vi "_Core(client).vi"(0 "XML config File Path":path=path "D:/work/Project support in lanzhou/OPCUA XML/xml/server config.xml", 1 "Server IP":string, 2 "client cert path(empty path)":path, 3 "timeout (5000 ms)":u32=5000, 4 "username/password":cluster{"username":string, "password":string}, 7 "error in (no error)":errorcluster, 9 "Op":T1) -> (8 "OPC UA data change event":refnum<user-event>, 10 "trusted Server certfications":path[](array[path]), 12 "server endpoint URL":string, 20 "OPC UA client refnum out":refnum<k21>, 27 "error out":errorcluster)   [LabVIEW 2014, in "OCPUA Client(UtilityMode).lvlib"]
uses:
  OCPUA Client(UtilityMode).lvlib
  _op(client).ctl
  <vilib>/OPCUA/NI OPC UA Client.lvlib
  OPCUA XML/OPCUA XML.lvlib
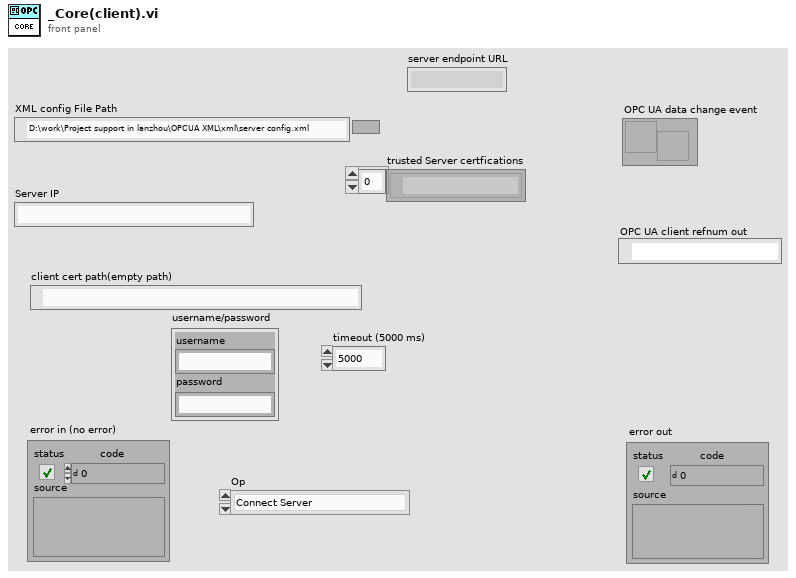
[diagram p1: front panel]
types:
  T1 = typedef "OCPUA Client(UtilityMode).lvlib/_op(client).ctl" = enum16{"Connect Server", "Get Client Refnum", "Disconnect Server"}
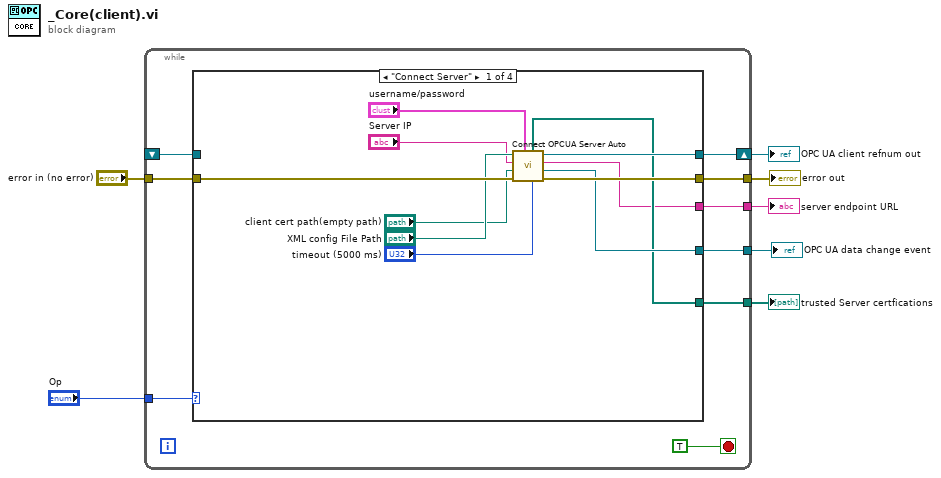
[diagram p0: block diagram]
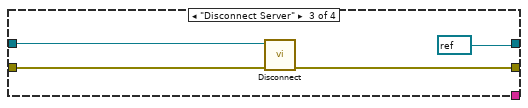
[diagram p3: hidden frame]
diagram:
  n1 = while {
    tunnel: "Op" -> [w15]
    shift-right: [w13] -> w4
    shift-left: _ -> [w14]
    tunnel: [w12] -> w5
    tunnel: "error in (no error)" -> [w11]
    tunnel: [w10] -> w3
    tunnel: [w9] -> w2
    tunnel: [w8] -> w1
    stop <- TRUE stop-if-true
    n2 = case shown="\"Connect Server\"" w15 {
      tunnel: w14 -> [_ w29 w31 w35]
      tunnel: [w25 w29 refnum<k21> refnum ("OPC UA client refnum out") w35] -> w13
      tunnel: [w27 w28 w32 w34] -> w12
      tunnel: w11 -> [w26 w28 w33 w34]
      tunnel: [w20 _ _ _] -> w10
      tunnel: [w19 _ _ _] -> w9
      tunnel: [w18 _ _ _] -> w8
      frame "Connect Server" {
        n3 = call "Connect OPCUA Server Auto.vi"("timeout (5000 ms)"="timeout (5000 ms)", "username/password"="username/password", "Error In"=w26, "client cert path(empty path)"="client cert path(empty path)", "Server IP"="Server IP", "XML config File Path"="XML config File Path") -> ("Error Out"=w27:errorcluster, "OPC UA data change event"=w20:refnum<user-event>, "server endpoint URL"=w18:string, "OPC UA client refnum"=w25:refnum<k21>, "trusted Server certfications"=w19:path[])  [unwired: 1 in]
      }
      frame "Get Client Refnum" {
      }
      frame "Disconnect Server" {
        n4 = call <vilib>:"Disconnect.vi"("error in (no error)"=w33, "OPC UA client refnum in"=w31) -> ("error out"=w32:errorcluster)  [unwired: 9 in]
      }
      frame Default {
      }
    }
  }
  "error out" <- w5
  "OPC UA client refnum out" <- w4
  "OPC UA data change event" <- w3
  "trusted Server certfications" <- w2
  "server endpoint URL" <- w1
